vi "Read ini File.vi"(8 "error in (no error)":errorcluster) -> (0 "error out":errorcluster, 3 "value":string)   [LabVIEW 2018]
uses:
  <vilib>/Utility/config.llb/Read Key (String).vi
  <vilib>/Utility/config.llb/NI_LVConfig.lvlib
panel:
  out "found?":bool
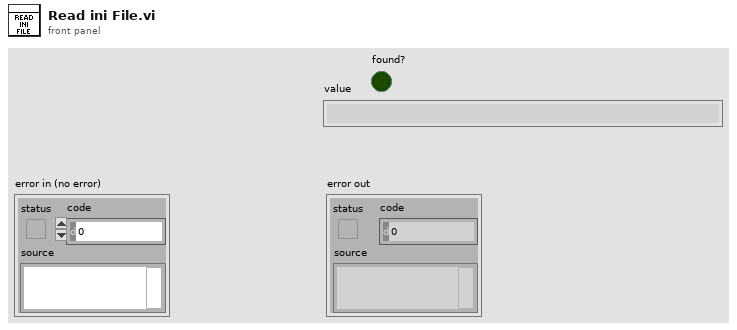
[diagram p1: front panel]
types:
  T1 = typedef "NI_LVConfig.lvlib/Config Data RefNum.ctl" = refnum<k1>
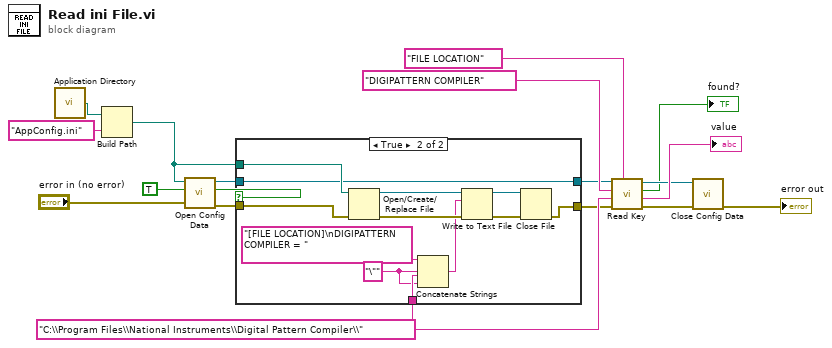
[diagram p0: block diagram]
diagram:
  w7 = "C:\\Program Files\\National Instruments\\Digital Pattern Compiler\\" ("default value")
  n1 = call <vilib>:"Application Directory.vi"() -> ("Application Directory"=w18:path)
  n2 = Build Path(base path=w18, name or relative path="AppConfig.ini") -> (appended path=w9:path)
  n3 = call <vilib>:"Open Config Data.vi"("error in (no error)"="error in (no error)", "create file if necessary (T)"=TRUE, "configuration file path"=w9) -> ("error out"=w8:errorcluster, "file created?"=w11:bool, "refnum"=w10:T1)  [unwired: 6 in]
  n4 = case shown="True" w11 {
    tunnel: w10 -> [w20 w21]
    tunnel: w9 -> [_ w31]
    tunnel: w8 -> [w19 w32]
    tunnel: w7 -> [_ w27]
    tunnel: [w19 w22] -> w6
    tunnel: [w20 w21] -> w5
    frame False {
    }
    frame True {
      w26 = "\"" ("string")
      n5 = Open/Create/Replace File(file path (use dialog)=w31, error in=w32) -> (refnum out=w29:refnum<file>, error out=w30:errorcluster)  [unwired: 4 in, 1 out]
      n6 = Concatenate Strings("[FILE LOCATION]\nDIGIPATTERN COMPILER = " ("text"), w26, w27, w26) -> (w25:string)
      n7 = Write to Text File(file (use dialog)=w29, text=w25, error in=w30) -> (refnum out=w23:refnum<file>, error out=w24:errorcluster)  [unwired: 1 in, 1 out]
      n8 = Close File(refnum=w23, error in=w24) -> (error out=w22:errorcluster)  [unwired: 1 out]
    }
  }
  n9 = call-poly <vilib>:"Read Key.vi"("section"="FILE LOCATION", "error in (no error)"=w6, "default value"=w7, "key"="DIGIPATTERN COMPILER", "refnum"=w5) -> ("error out"=w3:errorcluster, "value"=→"value":string, "found?"=→"found?":bool, "refnum out"=w4:T1)  [unwired: 3 in]
  n10 = call <vilib>:"Close Config Data.vi"("error in (no error)"=w3, "refnum"=w4) -> ("error out"=→"error out":errorcluster)  [unwired: 8 in, 1 out]
